vi "Read Geometry Definition Orient.vi"(8 "error in":errorcluster, 9 "Feature":string, 10 "Part Type":T1, 11 "Config Manager in":refnum<class "Config Manager Class.lvclass">) -> (0 "error out":errorcluster, 2 "Orient3d out":refnum<class "Orient3d Class.lvclass">, 3 "Config Manager out":refnum<class "Config Manager Class.lvclass">)   [LabVIEW 2011, in "Config Manager Class.lvclass"]
uses:
  Config Manager Class.lvclass
  Type Definitions/Part Type.ctl
  Orient3d Class/Orient3d Class.lvclass
  Config Manager Class.lvclass/Config Manager Class.ctl
  <vilib>/Utility/config.llb/Read Key (String).vi
  <vilib>/Utility/config.llb/NI_LVConfig.lvlib
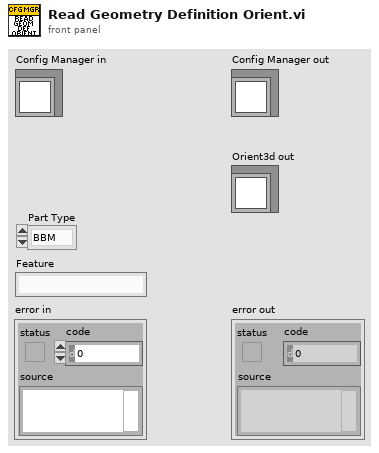
[diagram p1: front panel]
types:
  T1 = typedef "Part Type.ctl" = enum16{"BBM", "HDI", "BARE HDI", "GLUERESERVOIR", "STAMP_1", "STAMP_2", "STAMP_3", "STAMP_4", "STAMP_5", "WEIGHT_1", "WEIGHT_2", "WEIGHT_3", "WEIGHT_4", "WEIGHT_5", "WEIGHT_6", "WEIGHT_7", "WEIGHT_8", "PICKER_TOOL", "GRABER_TOOL"}
  T2 = typedef "NI_LVConfig.lvlib/Config Data RefNum.ctl" = refnum<k1>
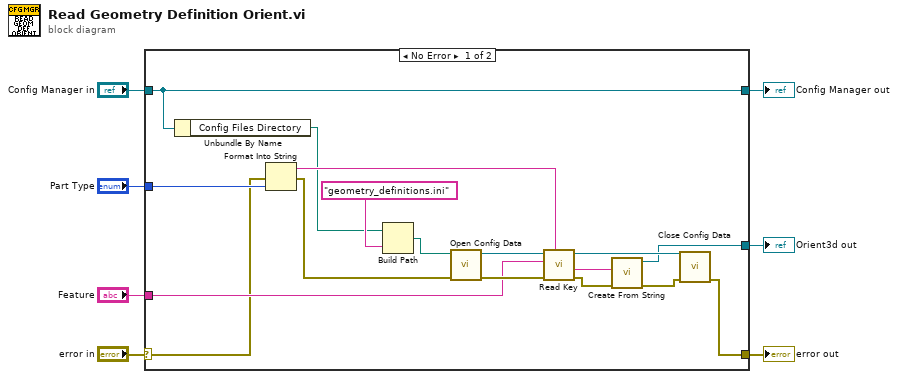
[diagram p0: block diagram]
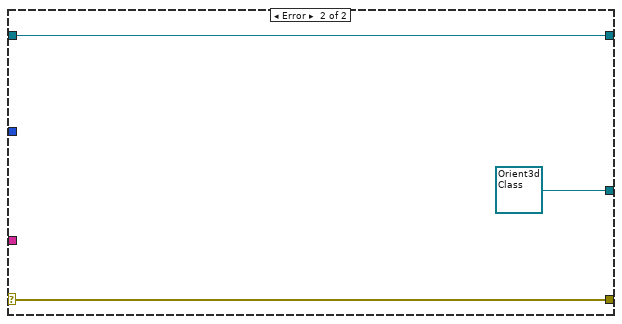
[diagram p2: hidden frame]
diagram:
  n1 = case shown="No Error" "error in" {
    selector: "error in" -> [w10 w27]
    tunnel: [w11 w27] -> w6
    tunnel: [w14 w26] -> w4
    tunnel: "Config Manager in" -> [w14 w26]
    tunnel: "Part Type" -> [w16 _]
    tunnel: "Feature" -> [w12 _]
    tunnel: [w8 refnum<class "Orient3d Class.lvclass"> refnum ("Orient3d out")] -> w1
    frame No Error {
      n2 = Unbundle By Name(w14) -> ("Config Files Directory"=w13:path)
      n3 = Format Into String(error in=w10, w16) -> (resulting string=w15:string, error out=w9:errorcluster)  [unwired: 2 in]
      n4 = Build Path(base path=w13, name or relative path="geometry_definitions.ini") -> (appended path=w23:path)
      n5 = call <vilib>:"Open Config Data.vi"("error in (no error)"=w9, "configuration file path"=w23) -> ("error out"=w21:errorcluster, "refnum"=w22:T2)  [unwired: 7 in, 1 out]
      n6 = call-poly <vilib>:"Read Key.vi"("section"=w15, "error in (no error)"=w21, "key"=w12, "refnum"=w22) -> ("error out"=w19:errorcluster, "value"=w20:string, "refnum out"=w18:T2)  [unwired: 4 in, 1 out]
      n7 = call "Create From String.vi"("error in"=w19, "Input String"=w20) -> ("error out"=w17:errorcluster, "Orient3d out"=w8:refnum<class "Orient3d Class.lvclass">)  [unwired: 8 in]
      n8 = call <vilib>:"Close Config Data.vi"("error in (no error)"=w17, "refnum"=w18) -> ("error out"=w11:errorcluster)  [unwired: 8 in, 1 out]
    }
    frame Error {
    }
  }
  "error out" <- w6
  "Config Manager out" <- w4
  "Orient3d out" <- w1
